vi "Get Port Status Response.vi"(8 "error in (no error)":errorcluster, 11 "Simulado in":refnum<class "Simulado.lvclass">) -> (0 "error out":errorcluster, 2 "Response":string, 3 "Simulado out":refnum<class "Simulado.lvclass">)   [LabVIEW 2020, in "Simulado.lvclass"]
uses:
  Simulado.lvclass
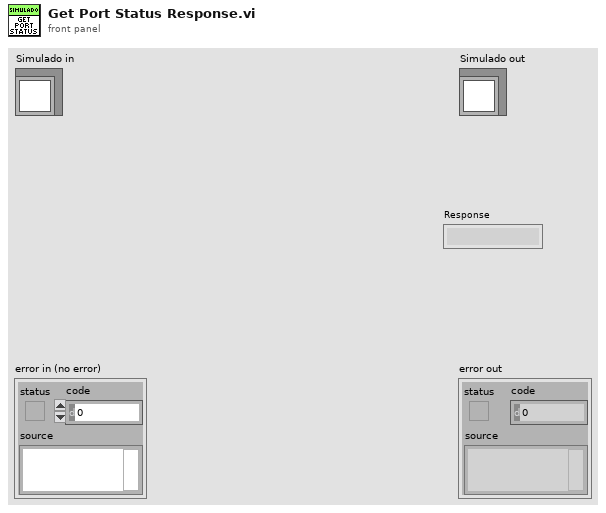
[diagram p1: front panel]
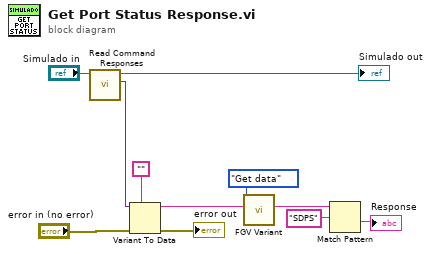
[diagram p0: block diagram]
diagram:
  n1 = call-dynamic "Read Command Responses.vi"("Simulado in"="Simulado in") -> ("Command Responses"=w9:variant, "Simulado out"=→"Simulado out":refnum<class "Simulado.lvclass">)  [unwired: 8 in, 1 out]
  n2 = Variant To Data(error in="error in (no error)", type="", Variant=w9) -> (data=w5:string, error out=→"error out":errorcluster)
  n3 = call "FGV Variant.vi"("Command"=w5, "Functions"=enum16{"Reset data", "Set data", "Get data"}."Get data") -> ("Response retrieved"=w1:string)  [unwired: 8 in, 1 out]
  n4 = Match Pattern(string=w1, regular expression="SDPS") -> (after substring=→"Response":string)  [unwired: 1 in, 3 out]
